vi "TIFF_Create_Metadata_General.vi"(8 "error in (no error)":errorcluster, 9 "XY resolution (nm)":string="125", 10 "Description":string="Embryo - GFP-Septin - RFP-Myosin", 11 "User":T2(ring)) -> (0 "error out":errorcluster, 1 "Metadata OUT":T1={"Date/Time"="15:07:2025 15:22:10", "System model"="Spinning Polar - 110", "Software version"="Labview - Polar_v2.0.lvproj", "Copyright"="IF - CNRS - AMU - CentraleMed - Mailfert - Honorine", "User"="Sophie Brasselet", "Description"="Embryo - GFP-Septin - RFP-Myosin", "X resolution"="125", "Y resolution"="125", "Resolution unit"="nm"}, 3 "Taggs":T1={"Date/Time"="/ifd/{ushort=306}", "System model"="/ifd/{ushort=272}", "Software version"="/ifd/{ushort=305}", "Copyright"="/ifd/{ushort=33432}", "User"="/ifd/{ushort=315}", "Description"="/ifd/{ushort=270}", "X resolution"="/ifd/{ushort=282}", "Y resolution"="/ifd/{ushort=283}", "Resolution unit"="/ifd/{ushort=296}"})   [LabVIEW 2025]
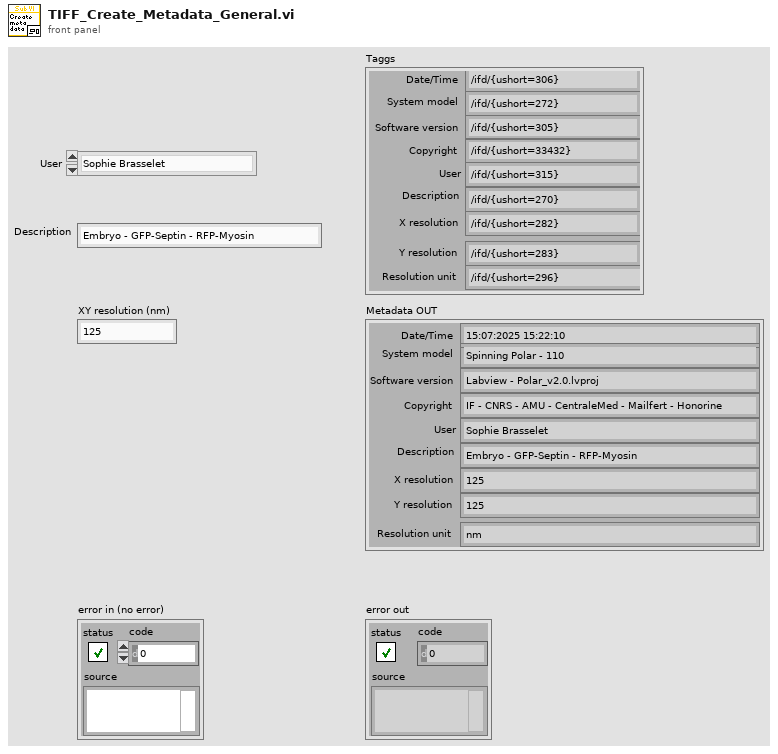
[diagram p1: front panel]
types:
  T1 = cluster{"Date/Time":string, "System model":string, "Software version":string, "Copyright":string, "User":string, "Description":string, "X resolution":string, "Y resolution":string, "Resolution unit":string}
  T2 = enum16{"Sophie Brasselet", "Jean-Jacques Honorine", "Sébastien Mailfert", "Manos Mavrakis"}
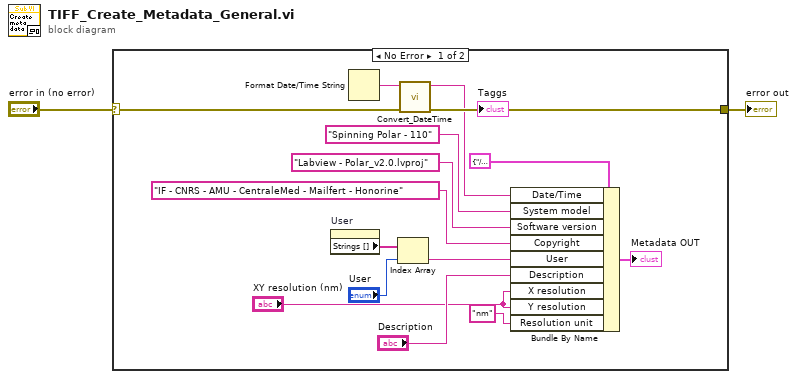
[diagram p0: block diagram]
diagram:
  n1 = case shown="No Error" "error in (no error)" {
    selector: "error in (no error)" -> [w5 w18]
    tunnel: [w4 w18] -> w2
    frame No Error {
      n2 = property on="User" class="Enum (strict)"() -> ("Strings []"=w17:string[])  [unwired: 2 in, 2 out]
      n3 = Format Date/Time String() -> (date/time string=w6:string)  [unwired: 3 in]
      n4 = Index Array(array=w17, index="User") -> (element=w9:string)
      n5 = call "Convert_DateTime.vi"("error in (no error)"=w5, "Date in (DD/MM/YYYY hh:mm:ss)"=w6) -> ("error out"=w4:errorcluster, "Date OUT (YYYY:MM:DD hh:mm:ss)"=w3:string)  [unwired: 8 in]
      n6 = Bundle By Name(cluster=T1 {"Date/Time"="/ifd/{ushort=306}", "System model"="/ifd/{ushort=272}", "Software version"="/ifd/{ushort=305}", "Copyright"="/ifd/{ushort=33432}", "User"="/ifd/{ushort=315}", "Description"="/ifd/{ushort=270}", "X resolution"="/ifd/{ushort=270}", "Y resolution"="/ifd/{ushort=270}", "Resolution unit"="/ifd/{ushort=270}"} ("Metadata"), "Date/Time"=w3, "System model"="Spinning Polar - 110", "Software version"="Labview - Polar_v2.0.lvproj", "Copyright"="IF - CNRS - AMU - CentraleMed - Mailfert - Honorine", "User"=w9, "Description"="Description", "X resolution"="XY resolution (nm)", "Y resolution"="XY resolution (nm)", "Resolution unit"="nm") -> (→"Metadata OUT":T1)
    }
    frame Error {
    }
  }
  "error out" <- w2
